vi "Main.vi"() -> ()   [LabVIEW 2026]
doc: "This template is for the Queued Message Handler design pattern.\n\nThe Event Handling Loop generates messages based on user interface actions.\n\nThe Message Handling Loop processes messages generated by the Event Handling Loop, or by other messages. The messages are string values, so new messages can be added easily to the Message Cases case structure in the Message Handling Loop. Each message cluster can also provide an optional value for Message Data, which is a variant that can be converted to whatever message-specific data is required."
uses:
  subVIs/DUT Info.ctl
  emea-tra-iPerf_bus_load_test/support/iperf3.Results.ctl
  subVIs/Proxy Config.ctl
  controls/UI Data.ctl
  support/Message Queue/Enqueue Message (Single).vi
  <vilib>/Utility/error.llb/Error Cluster From Error Code.vi
  <vilib>/ErrorRing/Error Ring.xnode
  support/Message Queue/Message Queue.lvlib
  support/User Event - Stop/User Event - Stop.lvlib
  emea-tra-iPerf_bus_load_test/iPerfTest.lvlib
panel:
  out "DASHBOARD":string[][](table)
  in  "LINK TEST":bool
  out "Link Speed Configured":u32(ring)=1 items=["100Mb/s"=1, "1000Mb/s"=2]
  in  "All Tests":bool
  in  "EXIT":bool
  out "Server results":T1
  out "Client results":T1
  out "config":string
  out "STATUS":string="\"Exit\" button pressed"
  in  "iperfTest":bool
  in  "LOG":bool
  in  "PING":bool
  in  "SETTINGS":T2(tab)=enum."Proxy Configuration"
  in  "XNET INTERFACE":string="ENET1"
  in  "PORT CONFIGURATION":T3(array[cluster])=[{"Name"="ENET1", "IPv4 Address"="192.168.1.3", "IPv4 Subnet Mask"="255.255.255.0", "IPv6 Address"="", "is tagged?"=FALSE, "VLAN ID"=0}]
  in  "SPEED":u32(ring)=2 items=["100Mb/s"=1, "1000Mb/s"=2]
  in  "SLEEP CAPABILITY":u32(ring) items=["Disabled", "Enabled"]
  in  "PROXY_CLIENT":bool
  in  "PROXY CONFIGURATION":T4[](array[typedef])=[{"PROTOCOL"="tcp", "DIRECTION"="outbound", "LISTEN ADRESS"="", "LISTEN PORT"=61000, "FWR DST ADRESS"="", "FWR DST PORT"=0, "FWR SRC ADRESS"="", "FWR SRC PORT"=0}, {"PROTOCOL"="tcp", "DIRECTION"="outbound", "LISTEN ADRESS"="", "LISTEN PORT"=61001, "FWR DST ADRESS"="", "FWR DST PORT"=0, "FWR SRC ADRESS"="", "FWR SRC PORT"=0}, {"PROTOCOL"="udp", "DIRECTION"="outbound", "LISTEN ADRESS"="127.0.0.1", "LISTEN PORT"=61001, "FWR DST ADRESS"="192.168.1.12", "FWR DST PORT"=61001, "FWR SRC ADRESS"="", "FWR SRC PORT"=62001}, {"PROTOCOL"="udp", "DIRECTION"="inbound", "LISTEN ADRESS"="192.168.1.3", "LISTEN PORT"=62001, "FWR DST ADRESS"="127.0.0.1", "FWR DST PORT"=62001, "FWR SRC ADRESS"="", "FWR SRC PORT"=61001}]
  in  "DUT Info":T5={"DUT IP"="192.168.1.12", "DUT Username"="Administrator", "DUT Password"="nitest", "DUT SSH PORT"=22, "DUT FWD TEST PORT"=62000, "DUT MAC ADDRESS"="02:00:08:38:2d:37"}
  in  "CONTINUOUS TEST":bool=TRUE
  in  "iPerf Test Parameters":T6={"CLIENT iPERF PORT"=61000, "Protocol"=enum."TCP", "Force traffic (UDP only)"=enum."1M", "DURATION iPERF TEST (s)"=10, "Stack mode"=enum."IP stack"}
  in  "Do Something Else <Replace Me>":bool
  # "These controls have associated \"Value Changed\" events configured in the Event Structure on the diagram.\n\nReplace them (and reconfigure the Event Structure) with the controls you need for your application."
  # "CONFIGURATION"
  # "RESULTS"
  # "This template is for the Queued Message Handler design pattern.\n\nSee the block diagram for more information on how to use this template."
  # "STATUS"
  # "CONTROL"
  # "TODO: Need to format these settings once defined which one we'll need"
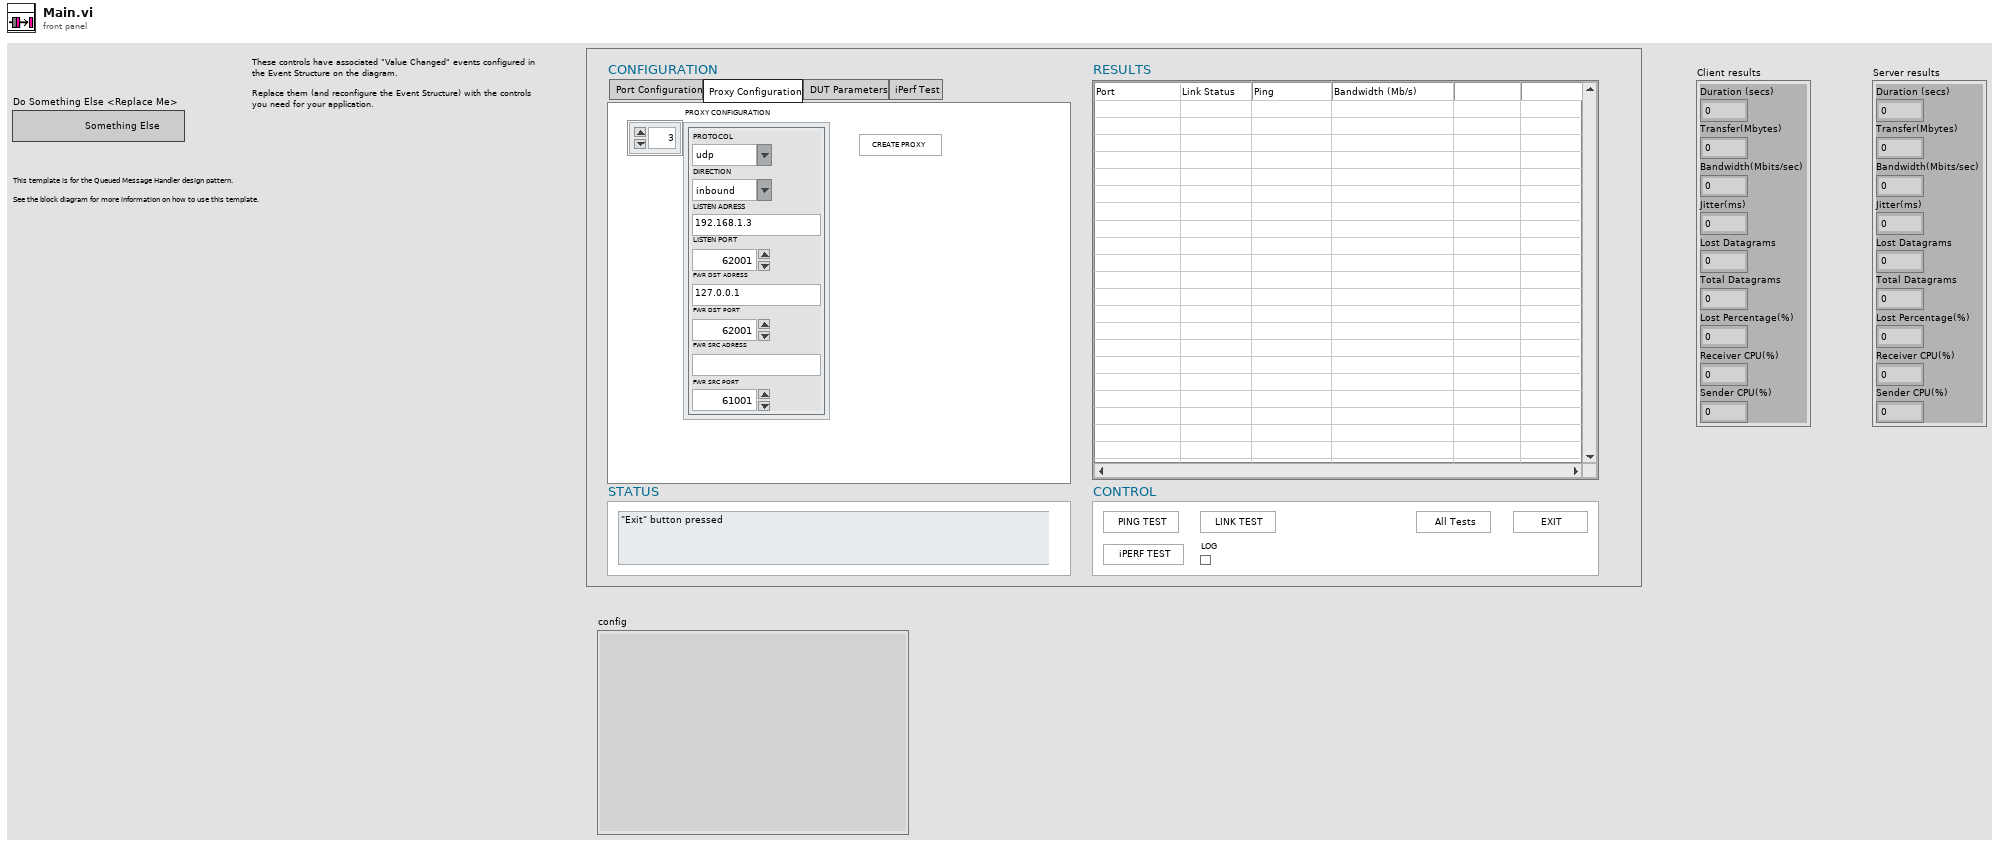
[diagram p1: front panel]
types:
  T1 = typedef "iPerfTest.lvlib/iperf3.Results.ctl" = cluster{"Duration (secs)":dbl, "Transfer(Mbytes)":dbl, "Bandwidth(Mbits/sec)":dbl, "Jitter(ms)":dbl, "Lost Datagrams":i32, "Total Datagrams":i32, "Lost Percentage(%)":dbl, "Receiver CPU(%)":dbl, "Sender CPU(%)":dbl}
  T2 = enum32{"Port Configuration", "Proxy Configuration", "DUT Parameters", "iPerf Test"}
  T3 = cluster{"Name":string, "IPv4 Address":string, "IPv4 Subnet Mask":string, "IPv6 Address":string, "is tagged?":bool, "VLAN ID":u16}[]
  T4 = typedef "Proxy Config.ctl" = cluster{"PROTOCOL":string, "DIRECTION":string, "LISTEN ADRESS":string, "LISTEN PORT":u16, "FWR DST ADRESS":string, "FWR DST PORT":u16, "FWR SRC ADRESS":string, "FWR SRC PORT":u16}
  T5 = typedef "DUT Info.ctl" = cluster{"DUT IP":string, "DUT Username":string, "DUT Password":string, "DUT SSH PORT":u16, "DUT FWD TEST PORT":u16, "DUT MAC ADDRESS":string}
  T6 = cluster{"CLIENT iPERF PORT":u16, "Protocol":enum16{"UDP", "TCP"}, "Force traffic (UDP only)":enum16{"1M", "10M", "20M", "30M", "40M", "50M", "100M", "500M", "1000M"}, "DURATION iPERF TEST (s)":u16, "Stack mode":enum16{"OS stack", "IP stack"}}
  T7 = typedef "UI Data.ctl" = cluster{"Boolean <Replace Me>":bool, "String <Replace Me>":string, "Numeric <Replace Me>":dbl, "Do Something Ref":refnum<vi>, "Do Something Else Ref":refnum<vi>, "Data Display Ref":refnum<vi>, "Exit Button Ref":refnum<vi>, "XNET INTERFACE":refnum<vi>, "Results":string}
  T8 = typedef "Message Queue.lvlib/All Message Queues.ctl" = cluster{"UI":refnum<queue>}
  T9 = cluster{"Name":string, "IPv4 Address":string, "IPv4 Subnet Mask":string, "IPv6 Address":string, "is tagged?":bool, "VLAN ID":u16}
  T10 = cluster{"TransmittedFrames":u32, "ReplyFrames":i32, "ICMP Echo ":string[]}
  T11 = typedef "Device Info.ctl" = cluster{"Interrupt Moderation":u32, "Jumbo Frames":u32, "Port Mode":u32, "PHY State":u32, "Sleep Capability Configured":u32, "Link Speed Configured":u32}
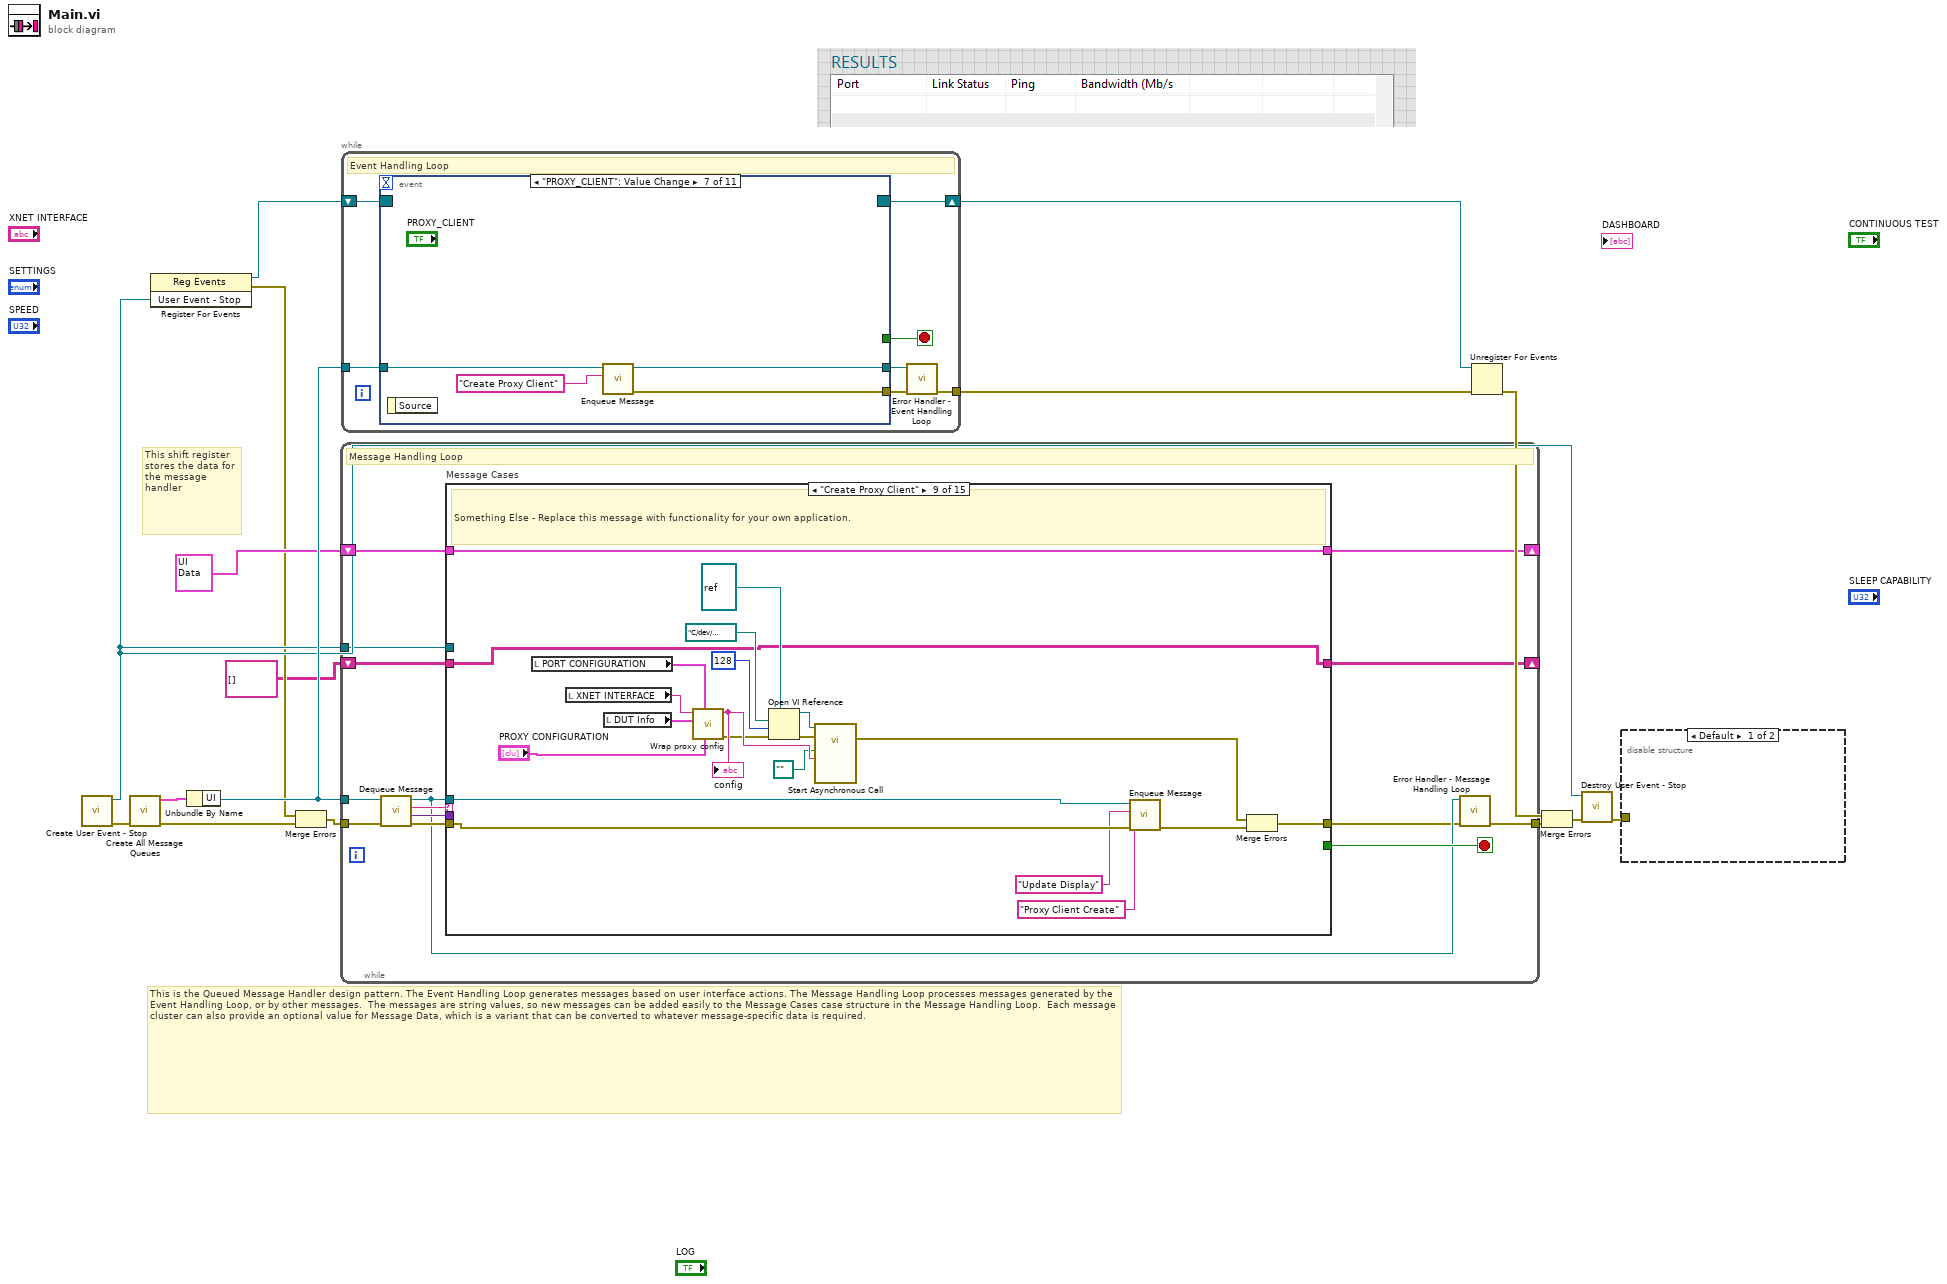
[diagram p0: block diagram]
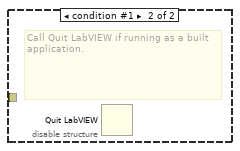
[diagram p2: hidden frame]
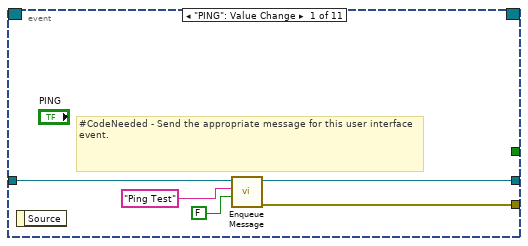
[diagram p3: hidden frame]
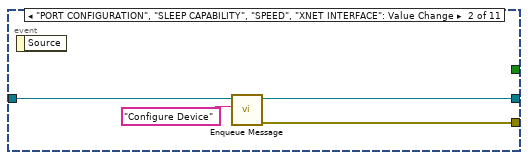
[diagram p4: hidden frame]
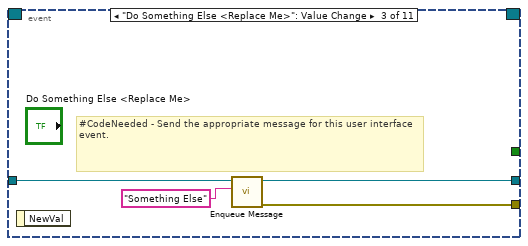
[diagram p5: hidden frame]
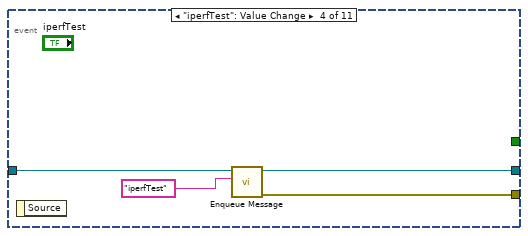
[diagram p6: hidden frame]
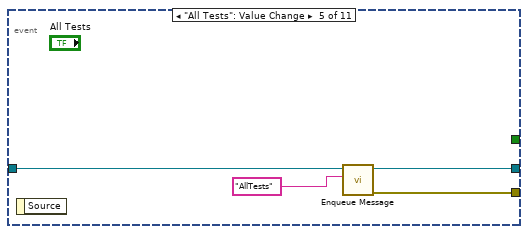
[diagram p7: hidden frame]
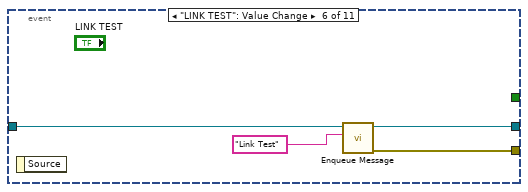
[diagram p8: hidden frame]
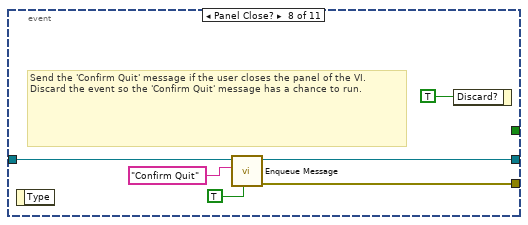
[diagram p9: hidden frame]
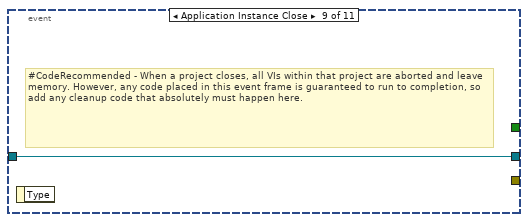
[diagram p10: hidden frame]
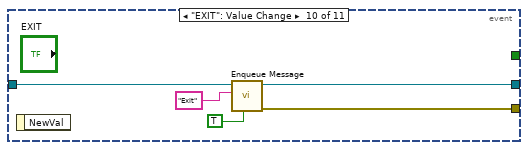
[diagram p11: hidden frame]
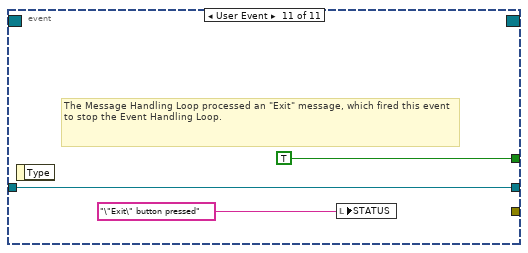
[diagram p12: hidden frame]
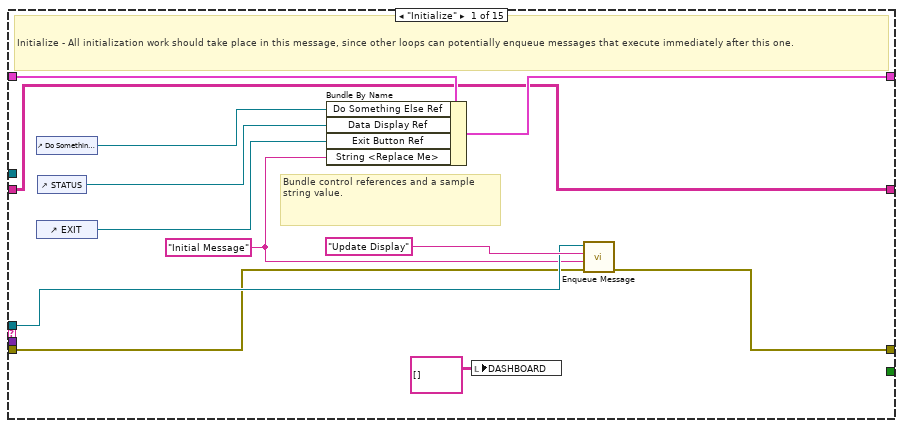
[diagram p13: hidden frame]
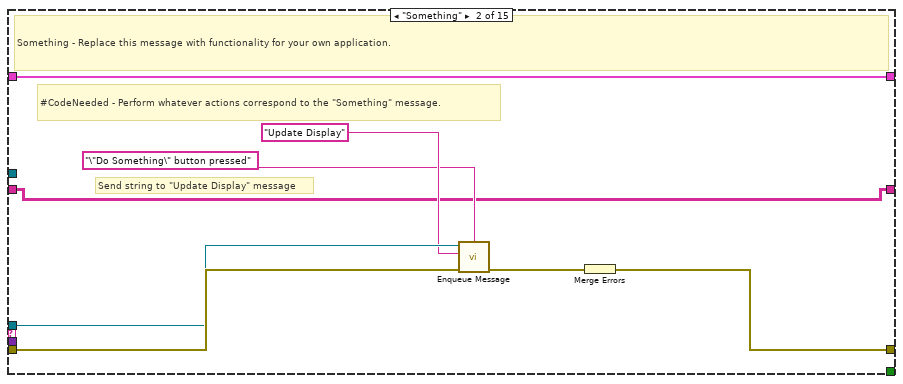
[diagram p14: hidden frame]
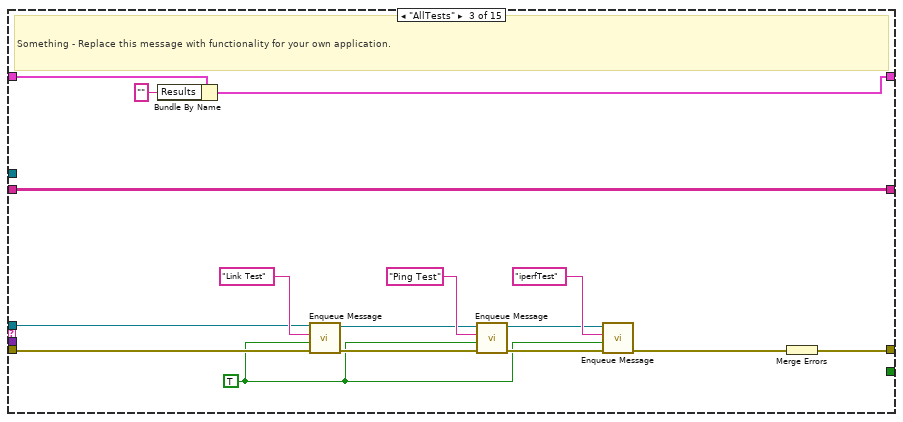
[diagram p15: hidden frame]
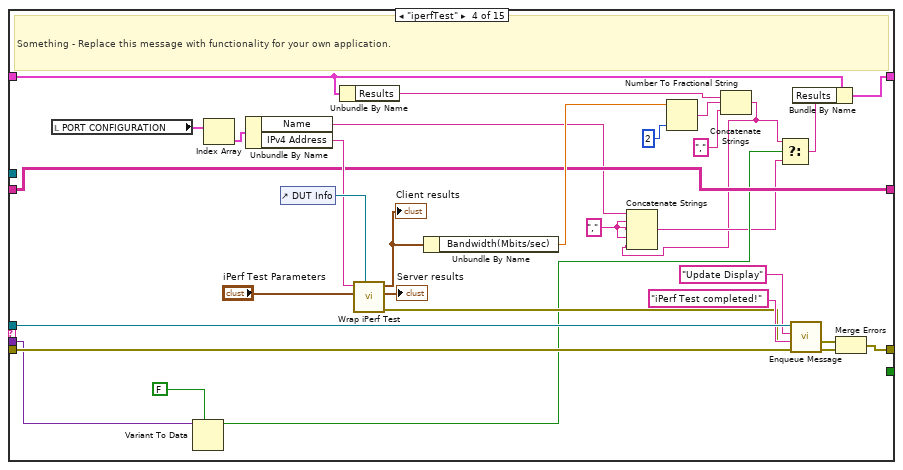
[diagram p16: hidden frame]
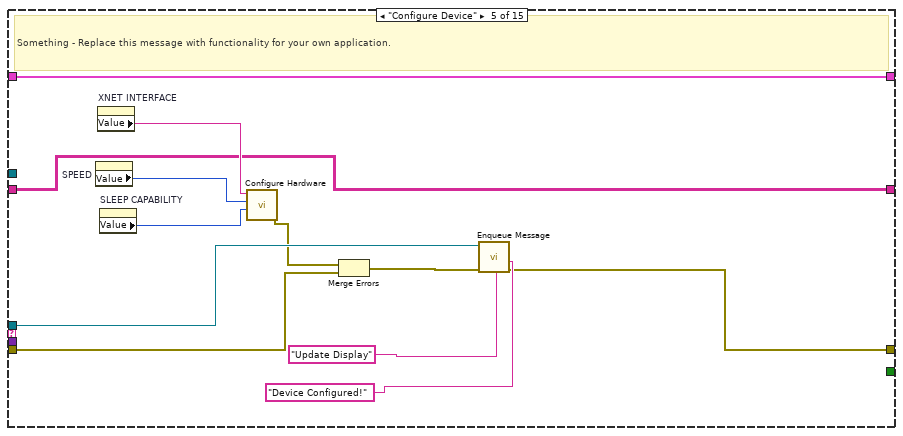
[diagram p17: hidden frame]
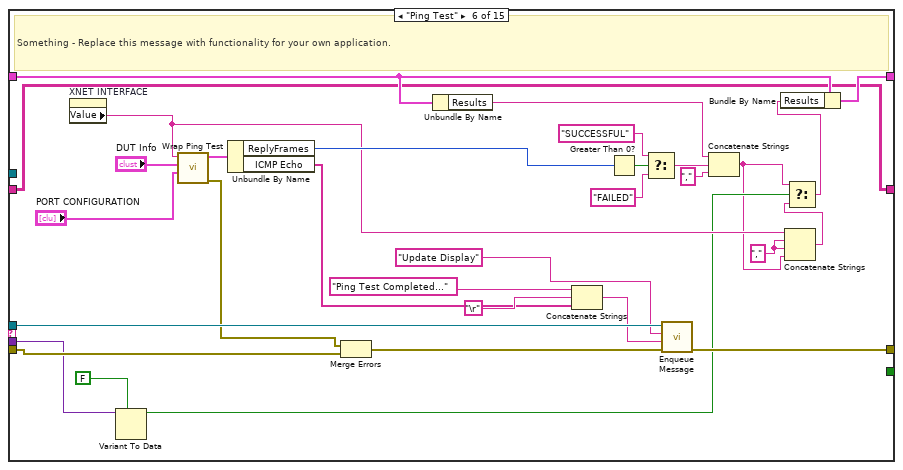
[diagram p18: hidden frame]
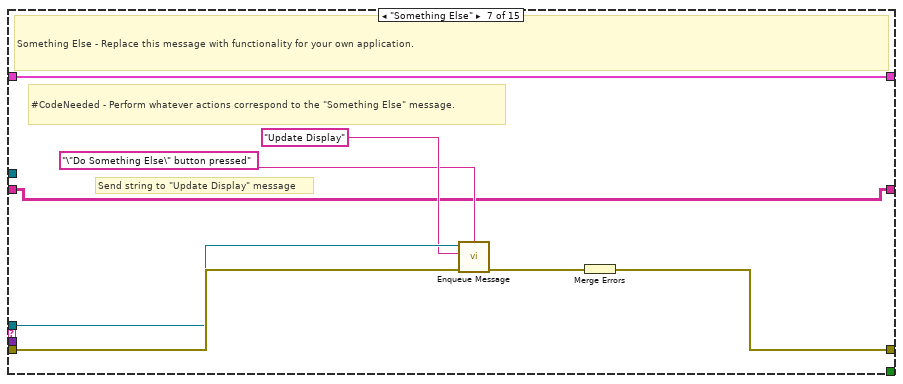
[diagram p19: hidden frame]
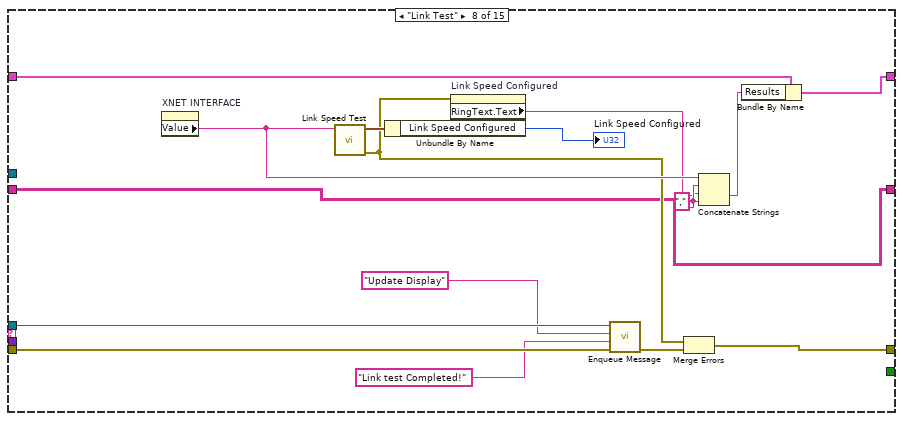
[diagram p20: hidden frame]
diagram:
  # "This is the Queued Message Handler design pattern. The Event Handling Loop generates messages based on user interface actions. The Message Handling Loop processes messages generated by the Event Handling Loop, or by other messages.  The messages are string values, so new messages can be added easily to the Message Cases case structure in the Message Handling Loop.  Each message cluster can also provide an optional value for Message Data, which is a variant that can be converted to whatever message-specific data is required."
  # "This shift register stores the data for the message handler"
  n1 = call "Create User Event - Stop.vi"() -> ("error out"=w12:errorcluster, "User Event - Stop"=w4:refnum<user-event>)  [unwired: 10 in]
  n2 = call "Create All Message Queues.vi"("error in (no error)"=w12) -> ("error out"=w16:errorcluster, "Message Queues out"=w15:T8)  [unwired: 9 in]
  n3 = register-events(w4) -> (reference out=w5:refnum<event-registration>, error out=w2:errorcluster)  [unwired: 2 in]
  n4 = Unbundle By Name(w15) -> ("UI"=w13:refnum<queue>)
  n5 = Merge Errors(w2, w16) -> (w3:errorcluster)
  n6 = while {
    tunnel: w13 -> [w23]
    shift-right: [w19] -> _
    shift-left: T7 {"Boolean <Replace Me>"=FALSE, "String <Replace Me>"="", "Numeric <Replace Me>"=0.0, "Do Something Ref"=refnum, "Do Something Else Ref"=refnum, "Data Display Ref"=refnum, "Exit Button Ref"=refnum, "XNET INTERFACE"=refnum, "Results"=""} ("Data Cluster") -> [w30]
    tunnel: w4 -> [w28]
    tunnel: w3 -> [w27]
    tunnel: [w21] -> w14
    shift-right: [w17] -> _
    shift-left: string[][] [] ("DASHBOARD") -> [w18]
    stop <- w29 stop-if-true
    # "Message Handling Loop"
    n7 = call "Dequeue Message.vi"("error in (no error)"=w27, "Message Queue"=w23) -> ("error out"=w26:errorcluster, "Message Data"=w24:variant, "Message"=w25:string, "dup Message Queue"=w22:refnum<queue>)  [unwired: 6 in]
    n8 = case "Message Cases" shown="\"Create Proxy Client\"" w25 {
      selector: w25 -> [_ _ _ _ _ _ _ _ _ _ _ _ _ _ w234]
      tunnel: w22 -> [w35 w46 w60 w93 w107 w139 w143 w160 w181 _ _ w212 _ w232 _]
      tunnel: w26 -> [w33 w48 w62 w95 w100 w135 w145 w162 w182 w199 w208 w216 w220 w225 _]
      tunnel: [w42 w49 w65 w96 w104 w134 w146 w163 w183 w200 w202 w214 w218 w228 w235] -> w20
      tunnel: w30 -> [w41 w50 w66 w77 w108 w121 w147 w154 w184 w191 w207 w215 w219 w231 w236]
      tunnel: [w40 w50 w58 w83 w108 w122 w147 w156 w184 w188 w207 w215 w219 w231 w236] -> w19
      tunnel: [_ _ _ _ _ _ _ _ _ _ _ _ _ TRUE _] -> w29
      tunnel: w24 -> [_ _ _ w73 _ w115 _ _ _ w198 w206 _ _ w222 _]
      tunnel: w28 -> [_ _ _ _ _ _ _ _ _ _ _ _ _ w227 _]
      tunnel: w18 -> [w32 w43 w53 w75 w97 w117 w140 w148 w168 w190 w201 w209 w217 w221 w233]
      tunnel: [w32 w43 w53 w75 w97 w117 w140 w148 w168 w185 w201 w209 w217 w221 w233] -> w17
      frame "Initialize" {
        w34 = "Initial Message" ("Initial Message")
        # "Bundle control references and a sample string value."
        # "Initialize - All initialization work should take place in this message, since other loops can potentially enqueue messages that execute immediately after this one."
        n9 = control-ref of="Do Something Else <Replace Me>"() -> (w39:refnum<vi>)
        n10 = control-ref of="EXIT"() -> (w37:refnum<vi>)
        n11 = control-ref of="STATUS"() -> (w38:refnum<vi>)
        n12 = Bundle By Name(cluster=w41, "Do Something Else Ref"=w39, "Data Display Ref"=w38, "Exit Button Ref"=w37, "String <Replace Me>"=w34) -> (w40:T7)
        n13 = local write "DASHBOARD"(string[][] [] ("DASHBOARD")) -> ()
        n14 = call-poly "Enqueue Message.vi"("error in (no error)"=w33, "Message Data"=w34, "Message"="Update Display", "Message Queue"=w35) -> ("error out"=w42:errorcluster)  [unwired: 6 in, 1 out]
      }
      frame "Something" {
        # "Send string to \"Update Display\" message"
        # "#CodeNeeded - Perform whatever actions correspond to the \"Something\" message."
        # "Something - Replace this message with functionality for your own application."
        n15 = call-poly "Enqueue Message.vi"("error in (no error)"=w48, "Message Data"="\"Do Something\" button pressed" ("\"Do Something\" button pressed"), "Message"="Update Display", "Message Queue"=w46) -> ("error out"=w47:errorcluster)  [unwired: 6 in, 1 out]
        n16 = Merge Errors(w47) -> (w49:errorcluster)
      }
      frame "AllTests" {
        w51 = TRUE
        # "Something - Replace this message with functionality for your own application."
        n17 = Bundle By Name(cluster=w66, "Results"="") -> (w58:T7)
        n18 = call-poly "Enqueue Message.vi"("error in (no error)"=w62, "Message Data"=w51, "Message"="Link Test", "Message Queue"=w60) -> ("error out"=w61:errorcluster, "dup Message Queue"=w59:refnum<queue>)  [unwired: 6 in]
        n19 = call-poly "Enqueue Message.vi"("error in (no error)"=w61, "Message Data"=w51, "Message"="Ping Test", "Message Queue"=w59) -> ("error out"=w55:errorcluster, "dup Message Queue"=w54:refnum<queue>)  [unwired: 6 in]
        n20 = call-poly "Enqueue Message.vi"("error in (no error)"=w55, "Message Data"=w51, "Message"="iperfTest", "Message Queue"=w54) -> ("error out"=w52:errorcluster)  [unwired: 6 in, 1 out]
        n21 = Merge Errors(w52) -> (w65:errorcluster)
      }
      frame "iperfTest" {
        w68 = "," ("string")
        # "Something - Replace this message with functionality for your own application."
        n22 = local read "PORT CONFIGURATION"() -> (w88:T3)
        n23 = Variant To Data(type=FALSE, Variant=w73) -> (data=w72:bool)  [unwired: 1 in, 1 out]
        n24 = Index Array(array=w88) -> (element=w87:T9)  [unwired: 1 in]
        n25 = Unbundle By Name(w87) -> ("Name"=w69:string, "IPv4 Address"=w85:string)
        n26 = control-ref of="DUT Info"() -> (w89:refnum<vi>)
        n27 = Unbundle By Name(w77) -> ("Results"=w76:string)
        n28 = call "Wrap iPerf Test.vi"("DUT Settings Ref"=w89, "iPerf Test Parameters"="iPerf Test Parameters", "Client_adapter_IP_remote"=w85) -> ("error out"=w90:errorcluster, "Server results"=→"Server results":T1, "Client results"=w82:T1)  [unwired: 6 in]
        "Client results" <- w82
        n29 = Unbundle By Name(w82) -> ("Bandwidth(Mbits/sec)"=w81:dbl)
        n30 = Number To Fractional String(number=w81, precision (6)=i16 2) -> (F-format string=w78:string)  [unwired: 2 in]
        n31 = Concatenate Strings(w76, w78, "," ("string")) -> (w67:string)
        n32 = Concatenate Strings(w69, w68, w68, w68, w67) -> (w71:string)
        n33 = Select(t=w67, s=w72, f=w71) -> (s? t:f=w70:string)
        n34 = call-poly "Enqueue Message.vi"("error in (no error)"=w95, "Message Data"="iPerf Test completed!" ("\"Do Something\" button pressed"), "Message"="Update Display", "Message Queue"=w93) -> ("error out"=w94:errorcluster)  [unwired: 6 in, 1 out]
        n35 = Bundle By Name(cluster=w77, "Results"=w70) -> (w83:T7)
        n36 = Merge Errors(w90, w94) -> (w96:errorcluster)
      }
      frame "Configure Device" {
        # "Something - Replace this message with functionality for your own application."
        n37 = property on="SPEED" class="Ring (strict)"() -> ("Value"=w103:u32)  [unwired: 2 in, 2 out]
        n38 = property on="XNET INTERFACE" class="Str"() -> ("Value"=w102:string)  [unwired: 2 in, 2 out]
        n39 = property on="SLEEP CAPABILITY" class="Ring (strict)"() -> ("Value"=w101:u32)  [unwired: 2 in, 2 out]
        n40 = call "Configure Hardware.vi"("Sleep Capability"=w101, "Link Speed"=w103, "XNET Interface"=w102) -> ("error out"=w99:errorcluster)  [unwired: 6 in, 2 out]
        n41 = Merge Errors(w99, w100) -> (w98:errorcluster)
        n42 = call-poly "Enqueue Message.vi"("error in (no error)"=w98, "Message Data"="Device Configured!" ("\"Do Something\" button pressed"), "Message"="Update Display", "Message Queue"=w107) -> ("error out"=w104:errorcluster)  [unwired: 6 in, 1 out]
      }
      frame "Ping Test" {
        w110 = "," ("string")
        # "Something - Replace this message with functionality for your own application."
        n43 = property on="XNET INTERFACE" class="Str"() -> ("Value"=w114:string)  [unwired: 2 in, 2 out]
        n44 = Variant To Data(type=FALSE, Variant=w115) -> (data=w113:bool)  [unwired: 1 in, 1 out]
        n45 = call "Wrap Ping Test.vi"("PORT CONFIGURATION"="PORT CONFIGURATION", "DUT Info"="DUT Info", "Interface Name"=w114) -> ("error out"=w136:errorcluster, "PingResults"=w131:T10)  [unwired: 7 in]
        n46 = Unbundle By Name(w131) -> ("ReplyFrames"=w123:i32, "ICMP Echo"=w130:string[])
        n47 = Merge Errors(w136, w135) -> (w133:errorcluster)
        n48 = Unbundle By Name(w121) -> ("Results"=w120:string)
        n49 = Concatenate Strings("Ping Test Completed..." ("\"Do Something\" button pressed"), "\r", w130) -> (w127:string)
        n50 = Greater Than 0?(x=w123) -> (x > 0?=w126:bool)
        n51 = Select(t="SUCCESSFUL" ("Message"), s=w126, f="FAILED" ("Message")) -> (s? t:f=w119:string)
        n52 = call-poly "Enqueue Message.vi"("error in (no error)"=w133, "Message Data"=w127, "Message"="Update Display", "Message Queue"=w139) -> ("error out"=w134:errorcluster)  [unwired: 6 in, 1 out]
        n53 = Concatenate Strings(w120, w119, "," ("string")) -> (w109:string)
        n54 = Concatenate Strings(w114, w110, w110, w109) -> (w112:string)
        n55 = Select(t=w109, s=w113, f=w112) -> (s? t:f=w111:string)
        n56 = Bundle By Name(cluster=w121, "Results"=w111) -> (w122:T7)
      }
      frame "Something Else" {
        # "Send string to \"Update Display\" message"
        # "#CodeNeeded - Perform whatever actions correspond to the \"Something Else\" message."
        # "Something Else - Replace this message with functionality for your own application."
        n57 = call-poly "Enqueue Message.vi"("error in (no error)"=w145, "Message Data"="\"Do Something Else\" button pressed" ("\"Do Something Else\" button pressed"), "Message"="Update Display", "Message Queue"=w143) -> ("error out"=w144:errorcluster)  [unwired: 6 in, 1 out]
        n58 = Merge Errors(w144) -> (w146:errorcluster)
      }
      frame "Link Test" {
        w155 = "," ("string")
        n59 = property on="XNET INTERFACE" class="Str"() -> ("Value"=w153:string)  [unwired: 2 in, 2 out]
        n60 = call "Link Speed Test.vi"("XNET Interface"=w153) -> ("error out"=w149:errorcluster, "DUT Info"=w157:T11)  [unwired: 9 in]
        n61 = Unbundle By Name(w157) -> ("Link Speed Configured"=→"Link Speed Configured":u32)
        n62 = property on="Link Speed Configured" class="Ring (strict)"(error in=w149) -> ("RingText.Text"=w150:string)  [unwired: 1 in, 2 out]
        n63 = call-poly "Enqueue Message.vi"("error in (no error)"=w162, "Message Data"="Link test Completed!" ("\"Do Something Else\" button pressed"), "Message"="Update Display", "Message Queue"=w160) -> ("error out"=w161:errorcluster)  [unwired: 6 in, 1 out]
        n64 = Merge Errors(w149, w161) -> (w163:errorcluster)
        n65 = Concatenate Strings(w153, w155, w150, w155) -> (w152:string)
        n66 = Bundle By Name(cluster=w154, "Results"=w152) -> (w156:T7)
      }
      frame "Create Proxy Client" {
        # "Something Else - Replace this message with functionality for your own application."
        n67 = local read "PORT CONFIGURATION"() -> (w173:T3)
        n68 = local read "XNET INTERFACE"() -> (w175:string)
        n69 = local read "DUT Info"() -> (w174:T5)
        n70 = call "Wrap proxy config.vi"("PROXY CONFIGURATION"="PROXY CONFIGURATION", "PORT CONFIGURATION"=w173, "DUT Info"=w174, "XNET INTERFACE"=w175) -> ("error out"=w171:errorcluster, "config"=w172:string)  [unwired: 6 in]
        "config" <- w172
        n71 = Open VI Reference(type specifier VI Refnum (for type only)=refnum<vi> refnum, vi path=path "C:/dev/automotive-interface-plugins/src/labview/auto-eth-generation/QMH/subVIs/proxy_for_client_plugin.vi", options=128, error in (no error)=w171) -> (vi reference=w166:refnum<vi>, error out=w165:errorcluster)  [unwired: 2 in]
        n72 = call-by-ref "Start Asynchronous Call"(reference=w166, error in=w165, "Config"=w172, "file path (use dialog)"=path "") -> (error out=w169:errorcluster)  [unwired: 10 in, 1 out]
        n73 = call-poly "Enqueue Message.vi"("error in (no error)"=w182, "Message Data"="Proxy Client Create" ("\"Do Something Else\" button pressed"), "Message"="Update Display", "Message Queue"=w181) -> ("error out"=w170:errorcluster)  [unwired: 6 in, 1 out]
        n74 = Merge Errors(w169, w170) -> (w183:errorcluster)
      }
      frame "Update Display" {
        # "#CodeRecommended - If you wish to decouple the Message Handling Loop from your user interface, consider creating User Events (like the \"Stop\" event in this VI) to message the Event Handling Loop whenever the user interface needs updating."
        # "Update Display - Convert the message data to a string to display in the Data Display indicator."
        n75 = Variant To Data(error in=w199, type="", Variant=w198) -> (data=→"STATUS":string, error out=w196:errorcluster)
        n76 = Unbundle By Name(w191) -> ("Results"=w192:string)
        n77 = Spreadsheet String To Array(delimiter (Tab)=",", format string="%s", spreadsheet string=w192, array type (2D Dbl)=string[][] [[""]] ("DASHBOARD")) -> (array=w189:string[][])
        n78 = Insert Into Array(array=w190, new element=w189) -> (w185:string[][])  [unwired: 2 in]
        n79 = Merge Errors(w196) -> (w200:errorcluster)
        n80 = Bundle By Name(cluster=w191, "Results"="") -> (w188:T7)
        n81 = local write "DASHBOARD"(w185) -> ()
      }
      frame "Error" {
        # "#CodeRecommended - If you ever change the name of this \"Error\" message, you'll need to update the name in the Check Loop Error.vi as well."
        # "#CodeRecommended - Consider creating a system for logging errors in some way. These errors are for notification purposes only. Handling of specific errors should be performed in the message frames that generated the error."
        # "Error - Display an error dialog. This message is sent by the \"Error Handler\" VIs at the end of other loops in this application."
        n82 = Variant To Data(error in=w208, type=errorcluster {"status"=FALSE, "code"=0, "source"=""} ("error constant"), Variant=w206) -> (data=w204:errorcluster, error out=w203:errorcluster)
        n83 = call <vilib>:"Simple Error Handler.vi"("error in (no error)"=w204) -> ()  [unwired: 4 in, 5 out]
        n84 = Merge Errors(w203) -> (w202:errorcluster)
      }
      frame "Confirm Quit" {
        # "#CodeNeeded - If you want to provide an \"Are you sure\" dialog (or some other notification) before the application exits, place that code here. This message is typically sent from a Panel Close? event."
        # "Confirm Quit - Message that can confirm whether or not the user wants to exit the application."
        n85 = call-poly "Enqueue Message.vi"("Priority Message? (F)"=TRUE, "error in (no error)"=w216, "Message"="Exit", "Message Queue"=w212) -> ("error out"=w213:errorcluster)  [unwired: 6 in, 1 out]
        n86 = Merge Errors(w213) -> (w214:errorcluster)
      }
      frame "---Copy This Frame---" {
        # "Duplicate this frame when creating new messages.  Change this comment in the duplicated frame to describe this message."
        n87 = Merge Errors(w220) -> (w218:errorcluster)
      }
      frame "Exit" {
        # "Stop the VI"
        # "Release the message queue reference"
        # "#CodeNeeded - Add any required cleanup code here. Note that if 'Exit' was called as a result of an error, an error dialog will be displayed. Add any custom error handling for an 'Exit' condition here as well."
        # "Exit - Exit the application."
        n88 = Variant To Data(type=errorcluster {"status"=FALSE, "code"=0, "source"=""} ("error constant"), Variant=w222) -> (data=w223:errorcluster)  [unwired: 1 in, 1 out]
        n89 = call <vilib>:"Simple Error Handler.vi"("error in (no error)"=w223) -> ()  [unwired: 4 in, 5 out]
        n90 = call "Fire User Event - Stop.vi"("User Event - Stop"=w227) -> ("error out"=w226:errorcluster)  [unwired: 10 in]
        n91 = Release Queue(queue=w232, error in (no error)=w225) -> (error out=w229:errorcluster)  [unwired: 1 in, 2 out]
        n92 = Merge Errors(w226, w229) -> (w228:errorcluster)
      }
      frame Default {
        # "'Default' case only runs if there is a message that isn't defined in any of the other cases.  Output a programming error."
        n93 = xnode "Error Ring"("parameter 0"=w234) -> ("error out"=w235:errorcluster)
      }
    }
    n94 = call "Error Handler - Message Handling Loop.vi"("error in (no error)"=w20, "Message Queue"=w22) -> ("dup error in"=w21:errorcluster)  [unwired: 8 in, 1 out]
  }
  n95 = while {
    tunnel: w13 -> [w250]
    shift-right: [w248] -> w9
    shift-left: w5 -> [w249]
    tunnel: [w244] -> w6
    stop <- w246 stop-if-true
    # "Event Handling Loop"
    n96 = event shown="[6] \"PROXY_CLIENT\": Value Change" {
      selector: w249 -> [_ _ _ _ _ _ _ _ _ _ _]
      dyn-events: [_ _ _ _ _ _ _ _ _ _ _] -> w248
      timeout: _ -> [_ _ _ _ _ _ _ _ _ _ _]
      tunnel: [_ _ _ _ _ _ _ _ _ _ TRUE ("Discard?")] -> w246
      tunnel: w250 -> [w255 w259 w263 w267 w271 w275 w279 w284 w286 w291 w294]
      tunnel: [w252 w256 w260 w264 w268 w272 w276 w283 _ w290 _] -> w247
      tunnel: [w254 w258 w262 w266 w270 w274 w278 w282 w286 w289 w294] -> w245
      event "PING": Value Change {
        # "#CodeNeeded - Send the appropriate message for this user interface event."
        n97 = event-data() -> ()  [unwired: 1 in, 1 out]
        n98 = call-poly "Enqueue Message.vi"("Message Data"=FALSE, "Message"="Ping Test", "Message Queue"=w255) -> ("error out"=w252:errorcluster, "dup Message Queue"=w254:refnum<queue>)  [unwired: 7 in]
      }
      event "PORT CONFIGURATION", "SLEEP CAPABILITY", "SPEED", "XNET INTERFACE": Value Change {
        n99 = event-data() -> ()  [unwired: 1 in, 1 out]
        n100 = call-poly "Enqueue Message.vi"("Message"="Configure Device", "Message Queue"=w259) -> ("error out"=w256:errorcluster, "dup Message Queue"=w258:refnum<queue>)  [unwired: 8 in]
      }
      event "Do Something Else <Replace Me>": Value Change {
        # "#CodeNeeded - Send the appropriate message for this user interface event."
        n101 = event-data() -> ()  [unwired: 1 in, 1 out]
        n102 = call-poly "Enqueue Message.vi"("Message"="Something Else", "Message Queue"=w263) -> ("error out"=w260:errorcluster, "dup Message Queue"=w262:refnum<queue>)  [unwired: 8 in]
      }
      event "iperfTest": Value Change {
        n103 = event-data() -> ()  [unwired: 1 in, 1 out]
        n104 = call-poly "Enqueue Message.vi"("Message"="iperfTest", "Message Queue"=w267) -> ("error out"=w264:errorcluster, "dup Message Queue"=w266:refnum<queue>)  [unwired: 8 in]
      }
      event "All Tests": Value Change {
        n105 = event-data() -> ()  [unwired: 1 in, 1 out]
        n106 = call-poly "Enqueue Message.vi"("Message"="AllTests", "Message Queue"=w271) -> ("error out"=w268:errorcluster, "dup Message Queue"=w270:refnum<queue>)  [unwired: 8 in]
      }
      event "LINK TEST": Value Change {
        n107 = event-data() -> ()  [unwired: 1 in, 1 out]
        n108 = call-poly "Enqueue Message.vi"("Message"="Link Test", "Message Queue"=w275) -> ("error out"=w272:errorcluster, "dup Message Queue"=w274:refnum<queue>)  [unwired: 8 in]
      }
      event "PROXY_CLIENT": Value Change {
        n109 = event-data() -> ()  [unwired: 1 in, 1 out]
        n110 = call-poly "Enqueue Message.vi"("Message"="Create Proxy Client", "Message Queue"=w279) -> ("error out"=w276:errorcluster, "dup Message Queue"=w278:refnum<queue>)  [unwired: 8 in]
      }
      event Panel Close? {
        # "Send the 'Confirm Quit' message if the user closes the panel of the VI. Discard the event so the 'Confirm Quit' message has a chance to run."
        n111 = event-data() -> ()  [unwired: 1 in, 1 out]
        n112 = call-poly "Enqueue Message.vi"("Priority Message? (F)"=TRUE, "Message"="Confirm Quit", "Message Queue"=w284) -> ("error out"=w283:errorcluster, "dup Message Queue"=w282:refnum<queue>)  [unwired: 7 in]
        n113 = event-data("Discard?"=TRUE) -> ()  [unwired: 1 in, 1 out]
      }
      event Application Instance Close {
        # "#CodeRecommended - When a project closes, all VIs within that project are aborted and leave memory. However, any code placed in this event frame is guaranteed to run to completion, so add any cleanup code that absolutely must happen here."
        n114 = event-data() -> ()  [unwired: 1 in, 1 out]
      }
      event "EXIT": Value Change {
        n115 = event-data() -> ()  [unwired: 1 in, 1 out]
        n116 = call-poly "Enqueue Message.vi"("Priority Message? (F)"=TRUE, "Message"="Exit", "Message Queue"=w291) -> ("error out"=w290:errorcluster, "dup Message Queue"=w289:refnum<queue>)  [unwired: 7 in]
      }
      event User Event {
        # "The Message Handling Loop processed an \"Exit\" message, which fired this event to stop the Event Handling Loop."
        n117 = event-data() -> ()  [unwired: 1 in, 1 out]
        n118 = local write "STATUS"("\"Exit\" button pressed" ("VI Stopped")) -> ()
      }
    }
    n119 = call "Error Handler - Event Handling Loop.vi"("error in (no error)"=w247, "Message Queue"=w245) -> ("dup error in"=w244:errorcluster)  [unwired: 8 in, 1 out]
  }
  n120 = Unregister For Events(event registration refnum=w9, error in=w6) -> (error out=w10:errorcluster)
  n121 = Merge Errors(w10, w14) -> (w11:errorcluster)
  n122 = call "Destroy User Event - Stop.vi"("error in (no error)"=w11, "User Event - Stop"=w4) -> ("error out"=w7:errorcluster)  [unwired: 9 in]
  n123 = disable-structure shown="Default" {
    disable-tunnel: w7 -> [_ _]
    frame condition #0 (active) {
    }
    frame condition #1 {
      # "Call Quit LabVIEW if running as a built application."
      n124 = Quit LabVIEW() -> ()  [unwired: 1 in]
    }
  }
